vi "Main.vi"() -> ()   [LabVIEW 2021] (continued)
                w2497 = T9 9 items=["刷新间隔", "波特率", "布尔1设置项", "布尔2设置项", "布尔3设置项", "布尔4设置项", "布尔5设置项", "显控1设置", "显控2设置", "显控3设置", "显控4设置", "显控5设置", "显控6设置", "显控7设置", "显控8设置", "显控9设置", "显控10设置", "显控11设置", "显控12设置", "设控1设置", "设控2设置", "设控3设置", "设控4设置", "设控5设置", "设控6设置", "设控7设置", "设控8设置", "曲线1设置", "曲线2设置", "曲线3设置", "曲线4设置", "曲线5设置", "曲线6设置", "曲线7设置", "曲线8设置", "曲线9设置", "曲线10设置", "曲线11设置", "曲线12设置", "曲线13设置", "曲线14设置", "曲线15设置", "曲线16设置", "ID值"] ("DataInitDef")
                w2496 = T9 10 items=["刷新间隔", "波特率", "布尔1设置项", "布尔2设置项", "布尔3设置项", "布尔4设置项", "布尔5设置项", "显控1设置", "显控2设置", "显控3设置", "显控4设置", "显控5设置", "显控6设置", "显控7设置", "显控8设置", "显控9设置", "显控10设置", "显控11设置", "显控12设置", "设控1设置", "设控2设置", "设控3设置", "设控4设置", "设控5设置", "设控6设置", "设控7设置", "设控8设置", "曲线1设置", "曲线2设置", "曲线3设置", "曲线4设置", "曲线5设置", "曲线6设置", "曲线7设置", "曲线8设置", "曲线9设置", "曲线10设置", "曲线11设置", "曲线12设置", "曲线13设置", "曲线14设置", "曲线15设置", "曲线16设置", "ID值"] ("DataInitDef")
                w2495 = T9 11 items=["刷新间隔", "波特率", "布尔1设置项", "布尔2设置项", "布尔3设置项", "布尔4设置项", "布尔5设置项", "显控1设置", "显控2设置", "显控3设置", "显控4设置", "显控5设置", "显控6设置", "显控7设置", "显控8设置", "显控9设置", "显控10设置", "显控11设置", "显控12设置", "设控1设置", "设控2设置", "设控3设置", "设控4设置", "设控5设置", "设控6设置", "设控7设置", "设控8设置", "曲线1设置", "曲线2设置", "曲线3设置", "曲线4设置", "曲线5设置", "曲线6设置", "曲线7设置", "曲线8设置", "曲线9设置", "曲线10设置", "曲线11设置", "曲线12设置", "曲线13设置", "曲线14设置", "曲线15设置", "曲线16设置", "ID值"] ("DataInitDef")
                w2494 = T9 18 items=["刷新间隔", "波特率", "布尔1设置项", "布尔2设置项", "布尔3设置项", "布尔4设置项", "布尔5设置项", "显控1设置", "显控2设置", "显控3设置", "显控4设置", "显控5设置", "显控6设置", "显控7设置", "显控8设置", "显控9设置", "显控10设置", "显控11设置", "显控12设置", "设控1设置", "设控2设置", "设控3设置", "设控4设置", "设控5设置", "设控6设置", "设控7设置", "设控8设置", "曲线1设置", "曲线2设置", "曲线3设置", "曲线4设置", "曲线5设置", "曲线6设置", "曲线7设置", "曲线8设置", "曲线9设置", "曲线10设置", "曲线11设置", "曲线12设置", "曲线13设置", "曲线14设置", "曲线15设置", "曲线16设置", "ID值"] ("DataInitDef")
                w2493 = T9 12 items=["刷新间隔", "波特率", "布尔1设置项", "布尔2设置项", "布尔3设置项", "布尔4设置项", "布尔5设置项", "显控1设置", "显控2设置", "显控3设置", "显控4设置", "显控5设置", "显控6设置", "显控7设置", "显控8设置", "显控9设置", "显控10设置", "显控11设置", "显控12设置", "设控1设置", "设控2设置", "设控3设置", "设控4设置", "设控5设置", "设控6设置", "设控7设置", "设控8设置", "曲线1设置", "曲线2设置", "曲线3设置", "曲线4设置", "曲线5设置", "曲线6设置", "曲线7设置", "曲线8设置", "曲线9设置", "曲线10设置", "曲线11设置", "曲线12设置", "曲线13设置", "曲线14设置", "曲线15设置", "曲线16设置", "ID值"] ("DataInitDef")
                w2504 = T9 7 items=["刷新间隔", "波特率", "布尔1设置项", "布尔2设置项", "布尔3设置项", "布尔4设置项", "布尔5设置项", "显控1设置", "显控2设置", "显控3设置", "显控4设置", "显控5设置", "显控6设置", "显控7设置", "显控8设置", "显控9设置", "显控10设置", "显控11设置", "显控12设置", "设控1设置", "设控2设置", "设控3设置", "设控4设置", "设控5设置", "设控6设置", "设控7设置", "设控8设置", "曲线1设置", "曲线2设置", "曲线3设置", "曲线4设置", "曲线5设置", "曲线6设置", "曲线7设置", "曲线8设置", "曲线9设置", "曲线10设置", "曲线11设置", "曲线12设置", "曲线13设置", "曲线14设置", "曲线15设置", "曲线16设置", "ID值"] ("DataInitDef")
                w2499 = T9 13 items=["刷新间隔", "波特率", "布尔1设置项", "布尔2设置项", "布尔3设置项", "布尔4设置项", "布尔5设置项", "显控1设置", "显控2设置", "显控3设置", "显控4设置", "显控5设置", "显控6设置", "显控7设置", "显控8设置", "显控9设置", "显控10设置", "显控11设置", "显控12设置", "设控1设置", "设控2设置", "设控3设置", "设控4设置", "设控5设置", "设控6设置", "设控7设置", "设控8设置", "曲线1设置", "曲线2设置", "曲线3设置", "曲线4设置", "曲线5设置", "曲线6设置", "曲线7设置", "曲线8设置", "曲线9设置", "曲线10设置", "曲线11设置", "曲线12设置", "曲线13设置", "曲线14设置", "曲线15设置", "曲线16设置", "ID值"] ("DataInitDef")
                w2503 = T9 14 items=["刷新间隔", "波特率", "布尔1设置项", "布尔2设置项", "布尔3设置项", "布尔4设置项", "布尔5设置项", "显控1设置", "显控2设置", "显控3设置", "显控4设置", "显控5设置", "显控6设置", "显控7设置", "显控8设置", "显控9设置", "显控10设置", "显控11设置", "显控12设置", "设控1设置", "设控2设置", "设控3设置", "设控4设置", "设控5设置", "设控6设置", "设控7设置", "设控8设置", "曲线1设置", "曲线2设置", "曲线3设置", "曲线4设置", "曲线5设置", "曲线6设置", "曲线7设置", "曲线8设置", "曲线9设置", "曲线10设置", "曲线11设置", "曲线12设置", "曲线13设置", "曲线14设置", "曲线15设置", "曲线16设置", "ID值"] ("DataInitDef")
                w2500 = T9 15 items=["刷新间隔", "波特率", "布尔1设置项", "布尔2设置项", "布尔3设置项", "布尔4设置项", "布尔5设置项", "显控1设置", "显控2设置", "显控3设置", "显控4设置", "显控5设置", "显控6设置", "显控7设置", "显控8设置", "显控9设置", "显控10设置", "显控11设置", "显控12设置", "设控1设置", "设控2设置", "设控3设置", "设控4设置", "设控5设置", "设控6设置", "设控7设置", "设控8设置", "曲线1设置", "曲线2设置", "曲线3设置", "曲线4设置", "曲线5设置", "曲线6设置", "曲线7设置", "曲线8设置", "曲线9设置", "曲线10设置", "曲线11设置", "曲线12设置", "曲线13设置", "曲线14设置", "曲线15设置", "曲线16设置", "ID值"] ("DataInitDef")
                w2502 = T9 16 items=["刷新间隔", "波特率", "布尔1设置项", "布尔2设置项", "布尔3设置项", "布尔4设置项", "布尔5设置项", "显控1设置", "显控2设置", "显控3设置", "显控4设置", "显控5设置", "显控6设置", "显控7设置", "显控8设置", "显控9设置", "显控10设置", "显控11设置", "显控12设置", "设控1设置", "设控2设置", "设控3设置", "设控4设置", "设控5设置", "设控6设置", "设控7设置", "设控8设置", "曲线1设置", "曲线2设置", "曲线3设置", "曲线4设置", "曲线5设置", "曲线6设置", "曲线7设置", "曲线8设置", "曲线9设置", "曲线10设置", "曲线11设置", "曲线12设置", "曲线13设置", "曲线14设置", "曲线15设置", "曲线16设置", "ID值"] ("DataInitDef")
                w2501 = T9 17 items=["刷新间隔", "波特率", "布尔1设置项", "布尔2设置项", "布尔3设置项", "布尔4设置项", "布尔5设置项", "显控1设置", "显控2设置", "显控3设置", "显控4设置", "显控5设置", "显控6设置", "显控7设置", "显控8设置", "显控9设置", "显控10设置", "显控11设置", "显控12设置", "设控1设置", "设控2设置", "设控3设置", "设控4设置", "设控5设置", "设控6设置", "设控7设置", "设控8设置", "曲线1设置", "曲线2设置", "曲线3设置", "曲线4设置", "曲线5设置", "曲线6设置", "曲线7设置", "曲线8设置", "曲线9设置", "曲线10设置", "曲线11设置", "曲线12设置", "曲线13设置", "曲线14设置", "曲线15设置", "曲线16设置", "ID值"] ("DataInitDef")
                n1889 = local read "控件配置文件"() -> (w2518:string[][])
                n1890 = local read "表格"() -> (w2517:string[][])
                n1891 = call "显示处理.vi"("项目"=w2500, "配置文件"=w2518, "表格"=w2517) -> ("显示"=→"显控9":string)  [unwired: 8 in]
                n1892 = call "显示处理.vi"("项目"=w2502, "配置文件"=w2518, "表格"=w2517) -> ("显示"=→"显控10":string)  [unwired: 8 in]
                n1893 = call "显示处理.vi"("项目"=w2503, "配置文件"=w2518, "表格"=w2517) -> ("显示"=→"显控8":string)  [unwired: 8 in]
                n1894 = call "显示处理.vi"("项目"=w2499, "配置文件"=w2518, "表格"=w2517) -> ("显示"=→"显控7":string)  [unwired: 8 in]
                n1895 = call "显示处理.vi"("项目"=w2501, "配置文件"=w2518, "表格"=w2517) -> ("显示"=→"显控11":string)  [unwired: 8 in]
                n1896 = call "显示处理.vi"("项目"=w2504, "配置文件"=w2518, "表格"=w2517) -> ("显示"=→"显控1":string)  [unwired: 8 in]
                n1897 = call "显示处理.vi"("项目"=w2497, "配置文件"=w2518, "表格"=w2517) -> ("显示"=→"显控3":string)  [unwired: 8 in]
                n1898 = call "显示处理.vi"("项目"=w2498, "配置文件"=w2518, "表格"=w2517) -> ("显示"=→"显控2":string)  [unwired: 8 in]
                n1899 = call "显示处理.vi"("项目"=w2496, "配置文件"=w2518, "表格"=w2517) -> ("显示"=→"显控4":string)  [unwired: 8 in]
                n1900 = call "显示处理.vi"("项目"=w2495, "配置文件"=w2518, "表格"=w2517) -> ("显示"=→"显控5":string)  [unwired: 8 in]
                n1901 = call "显示处理.vi"("项目"=w2494, "配置文件"=w2518, "表格"=w2517) -> ("显示"=→"显控12":string)  [unwired: 8 in]
                n1902 = call "显示处理.vi"("项目"=w2493, "配置文件"=w2518, "表格"=w2517) -> ("显示"=→"显控6":string)  [unwired: 8 in]
                n1903 = local read "控件配置文件"() -> (w2483:string[][])
                n1904 = local read "表格"() -> (w2484:string[][])
                n1905 = call "显示处理.vi"("项目"=w2485, "配置文件"=w2483, "表格"=w2484) -> ("显示"=w2482:string)  [unwired: 8 in]
                n1906 = call "显示处理.vi"("项目"=w2488, "配置文件"=w2483, "表格"=w2484) -> ("显示"=w2481:string)  [unwired: 8 in]
                n1907 = call "显示处理.vi"("项目"=w2487, "配置文件"=w2483, "表格"=w2484) -> ("显示"=w2480:string)  [unwired: 8 in]
                n1908 = call "显示处理.vi"("项目"=w2489, "配置文件"=w2483, "表格"=w2484) -> ("显示"=w2479:string)  [unwired: 8 in]
                n1909 = call "显示处理.vi"("项目"=w2490, "配置文件"=w2483, "表格"=w2484) -> ("显示"=w2478:string)  [unwired: 8 in]
                n1910 = call "显示处理.vi"("项目"=w2491, "配置文件"=w2483, "表格"=w2484) -> ("显示"=w2477:string)  [unwired: 8 in]
                n1911 = call "显示处理.vi"("项目"=w2492, "配置文件"=w2483, "表格"=w2484) -> ("显示"=w2476:string)  [unwired: 8 in]
                n1912 = call "显示处理.vi"("项目"=w2486, "配置文件"=w2483, "表格"=w2484) -> ("显示"=w2475:string)  [unwired: 8 in]
                n1913 = local write "设控6"(w2477) -> ()
                n1914 = local write "设控7"(w2476) -> ()
                n1915 = local write "设控1"(w2482) -> ()
                n1916 = local write "设控4"(w2479) -> ()
                n1917 = local write "设控8"(w2475) -> ()
                n1918 = local write "设控2"(w2481) -> ()
                n1919 = local write "设控3"(w2480) -> ()
                n1920 = local write "设控5"(w2478) -> ()
              }
            }
          }
        }
      }
      frame #3 {
        n1921 = disable-structure shown="启用" {
          frame Disabled {
          }
          frame Enabled {
          }
        }
      }
    }
    n1922 = Wait on Notification(notifier=w26) -> (error out=w27:errorcluster)  [unwired: 3 in, 3 out]
  }
  n1923 = Build Path(base path=w16, name or relative path="Config\\Config.ini" ("名称或相对路径")) -> (appended path=w15:path)
  n1924 = timed-loop {
    shift-right: [w2536] -> _
    shift-left: w24 -> [w2537]
    shift-right: [w2534] -> w3
    shift-left: errorcluster {"status"=FALSE, "code"=0, "source"=""} ("error constant") -> [w2535]
    tunnel: w15 -> [w2531]
    timing: w20 -> [_]
    timing-out: [_] -> w19
    shift-right: [w2529] -> w13
    shift-left: w10 -> [w2524]
    shift-right: [w2528] -> w12
    shift-left: w14 -> [w2530]
    tunnel: w7 -> [w2523]
    stop <- FALSE stop-if-true
    # "主程序通信VI状态机"
    n1925 = node-c288() -> ()  [unwired: 1 in, 1 out]
    n1926 = Increment(x="i1") -> (x+1=w2519:i32)
    n1927 = case shown="\"Process\"" w2537 {
      tunnel: [w2596 w2627 w2653 w2668 w2826 w2830 w2836] -> w2536
      tunnel: [w2597 FALSE ("停止循环？") FALSE ("停止循环？") FALSE ("停止循环？") TRUE ("停止循环？") FALSE ("停止循环？") FALSE ("布尔 2")] -> _
      tunnel: w2535 -> [_ w2640 w2659 _ w2823 w2832 w2837]
      tunnel: [w2590 w2638 w2650 _ w2825 w2831 w2837] -> w2534
      tunnel: "重新连接" -> [w2595 w2626 w2652 w2667 _ _ _]
      tunnel: w2519 -> [_ _ _ w2661 _ _ _]
      tunnel: w2531 -> [w2589 _ _ _ _ _ _]
      frame "Initialize", Default {
        w2591 = State."ERROR"  # 下一个状态
        w2597 = FALSE  # 停止循环？
        w2594 = State."ResetCAN"  # 下一个状态
        # "初始化－对应用程序进行初始化。"
        n1928 = Select(t=w2594, s=TRUE, f=State."Exit" ("下一个状态")) -> (s? t:f=w2592:T3)
        n1929 = flat-sequence {
          tunnel: w2589 -> [w2599]
          tunnel: [w2599] -> w2588
          tunnel: w2588 -> [w2609]
          tunnel: [w2611] -> w2590
          frame #0 {
            n1930 = for {
              N: 8 -> [_]
              i -> [w2601]
              n1931 = Add(x=81, y=w2601) -> (x+y=w2600:i32)
              n1932 = call "CAN Uninitialize.vi"("Channel"=w2600) -> ()  [unwired: 9 in, 2 out]
            }
          }
          frame #1 {
            w2603 = T9 1 items=["刷新间隔", "波特率", "布尔1设置项", "布尔2设置项", "布尔3设置项", "布尔4设置项", "布尔5设置项", "布尔6设置项", "布尔7设置项", "布尔8设置项", "显控1设置", "显控2设置", "显控3设置", "显控4设置", "显控5设置", "显控6设置", "显控7设置", "显控8设置", "显控9设置", "显控10设置", "显控11设置", "显控12设置", "设控1设置", "设控2设置", "设控3设置", "设控4设置", "设控5设置", "设控6设置", "设控7设置", "设控8设置", "曲线1设置", "曲线2设置", "曲线3设置", "曲线4设置", "曲线5设置", "曲线6设置", "曲线7设置", "曲线8设置", "曲线9设置", "曲线10设置", "曲线11设置", "曲线12设置", "曲线13设置", "曲线14设置", "曲线15设置", "曲线16设置", "曲线17设置", "曲线18设置", "曲线19设置", "曲线20设置", "曲线21设置", "曲线22设置", "曲线23设置", "曲线24设置", "曲线25设置", "曲线26设置", "曲线27设置", "曲线28设置", "曲线29设置", "曲线30设置", "曲线31设置", "曲线32设置", "曲线33设置", "曲线34设置", "曲线35设置", "曲线36设置", "曲线37设置", "曲线38设置", "曲线39设置", "曲线40设置", "曲线41设置", "曲线42设置", "曲线43设置", "曲线44设置", "曲线45设置", "曲线46设置", "曲线47设置", "曲线48设置", "曲线49设置", "曲线50设置", "曲线51设置", "曲线52设置", "曲线53设置", "曲线54设置", "曲线55设置", "曲线56设置", "曲线57设置", "曲线58设置", "曲线59设置", "曲线60设置", "曲线61设置", "曲线62设置", "曲线63设置", "曲线64设置", "ID值", "数据模式"] ("DataInitDef")
            w2604 = T9 0 items=["刷新间隔", "波特率", "布尔1设置项", "布尔2设置项", "布尔3设置项", "布尔4设置项", "布尔5设置项", "布尔6设置项", "布尔7设置项", "布尔8设置项", "显控1设置", "显控2设置", "显控3设置", "显控4设置", "显控5设置", "显控6设置", "显控7设置", "显控8设置", "显控9设置", "显控10设置", "显控11设置", "显控12设置", "设控1设置", "设控2设置", "设控3设置", "设控4设置", "设控5设置", "设控6设置", "设控7设置", "设控8设置", "曲线1设置", "曲线2设置", "曲线3设置", "曲线4设置", "曲线5设置", "曲线6设置", "曲线7设置", "曲线8设置", "曲线9设置", "曲线10设置", "曲线11设置", "曲线12设置", "曲线13设置", "曲线14设置", "曲线15设置", "曲线16设置", "曲线17设置", "曲线18设置", "曲线19设置", "曲线20设置", "曲线21设置", "曲线22设置", "曲线23设置", "曲线24设置", "曲线25设置", "曲线26设置", "曲线27设置", "曲线28设置", "曲线29设置", "曲线30设置", "曲线31设置", "曲线32设置", "曲线33设置", "曲线34设置", "曲线35设置", "曲线36设置", "曲线37设置", "曲线38设置", "曲线39设置", "曲线40设置", "曲线41设置", "曲线42设置", "曲线43设置", "曲线44设置", "曲线45设置", "曲线46设置", "曲线47设置", "曲线48设置", "曲线49设置", "曲线50设置", "曲线51设置", "曲线52设置", "曲线53设置", "曲线54设置", "曲线55设置", "曲线56设置", "曲线57设置", "曲线58设置", "曲线59设置", "曲线60设置", "曲线61设置", "曲线62设置", "曲线63设置", "曲线64设置", "ID值", "数据模式"] ("DataInitDef")
            w2606 = T12 0 items=["CONFIG"] ("Config Section")
            # "1、从配置文件中读取上一次的记录。"
            n1933 = call "Read ini.vi"("configuration file path"=w2609) -> ("数组"=w2605:string[][])  [unwired: 10 in]
            "配置文件" <- w2605
            n1934 = Index Array(array=w2605, index (row)=w2606, index (col)=w2604) -> (element=w2610:string)
            n1935 = Index Array(array=w2605, index (row)=w2606, index (col)=w2603) -> (element=w2608:string)
            n1936 = property on="刷新间隔" class="Str"("Value"=w2610) -> ()  [unwired: 2 in, 2 out]
            n1937 = Hexadecimal String To Number(string=w2608) -> (number=w2607:u32)  [unwired: 2 in, 1 out]
            n1938 = property on="波特率" class="Ring (严格)"("Value"=w2607) -> ()  [unwired: 2 in, 2 out]
          }
          frame #2 {
            # "2、初始化CAN"
            n1939 = while {
              tunnel: [w2621] -> w2611
              i -> [w2614]
              stop <- w2615 stop-if-true
              w2613 = u8 81 ("Channel")
              n1940 = Add(x=w2613, y=w2614) -> (x+y=w2612:i32)
              "CAN通道" <- w2612
              n1941 = call "CAN Initialize.vi"("Btr0Btr1"="波特率", "Channel"=w2612) -> ("error out"=w2621:errorcluster, "function return"=w2616:u32)  [unwired: 8 in]
              n1942 = Equal To 0?(x=w2616) -> (x = 0?=w2617:bool)
              n1943 = Greater?(x=w2613, y=7) -> (0:w2618:bool)
              n1944 = Or(x=w2618, y=w2617) -> (x .or. y?=w2615:bool)
            }
          }
        }
        n1945 = Select(t=w2591, s=w2595, f=w2592) -> (s? t:f=w2596:T3)
        n1946 = call <vilib>:"Application Directory.vi"() -> ("Application Directory"=w2587:path)
        n1947 = Path To String(path=w2587) -> (string=w2586:string)
        n1948 = Reverse String(1:w2586) -> (0:w2585:string)
        n1949 = Match Pattern(string=w2585, regular expression="\\" ("正则表达式")) -> (before substring=w2583:string)  [unwired: 1 in, 3 out]
        n1950 = Reverse String(1:w2583) -> (0:w2582:string)
        n1951 = property on="项目名" class="Str"("Caption.Text"=w2582) -> ()  [unwired: 2 in, 2 out]
      }
      frame "ResetCAN" {
        # "复位CAN模块，并读取CAN模块的状态"
        n1952 = local read "CAN通道"() -> (w2623:u8)
        n1953 = call "CAN Reset.vi"("error in (no error)"=w2640, "Channel"=w2623) -> ("error out"=w2639:errorcluster, "function return"=w2634:u32)  [unwired: 8 in]
        n1954 = call "CAN Get Status.vi"("error in (no error)"=w2639, "Channel"=w2623) -> ("error out"=w2638:errorcluster, "function return"=w2637:u32)  [unwired: 8 in]
        n1955 = Equal To 0?(x=w2634) -> (x = 0?=w2633:bool)
        n1956 = Equal To 0?(x=w2637) -> (x = 0?=w2632:bool)
        n1957 = And(x=w2633, y=w2632) -> (x .and. y?=w2624:bool)
        n1958 = Select(t=State."SetCAN" ("下一个状态"), s=w2624, f=State."ERROR" ("返回初始状态")) -> (s? t:f=w2630:T3)
        n1959 = Select(t=w2630, s=TRUE, f=State."Exit" ("返回初始状态")) -> (s? t:f=w2628:T3)
        n1960 = Select(t=State."ERROR" ("下一个状态"), s=w2626, f=w2628) -> (s? t:f=w2627:T3)
      }
      frame "SetCAN" {
        w2655 = State."ERROR"  # 下一个状态
        w2657 = State."Exit"  # 返回初始状态
        w2656 = State."Process"  # 初始状态
        # "设置CAN模块的参数"
        n1961 = local read "CAN通道"() -> (w2643:u8)
        n1962 = Select(t=w2656, s=TRUE, f=w2657) -> (s? t:f=w2654:T3)
        n1963 = call "CAN Get Value.vi"("BufferLength"=u32 4, "error in (no error)"=w2659, "Parameter"=u8 1, "Channel"=w2643) -> ("error out"=w2644:errorcluster)  [unwired: 4 in, 3 out]
        n1964 = Select(t=w2655, s=w2652, f=w2654) -> (s? t:f=w2653:T3)
        n1965 = call "CAN Set Value.vi"("BufferLength"=u32 1280, "error in (no error)"=w2644, "Parameter"=u8 3, "Channel"=w2643) -> ("error out"=w2645:errorcluster)  [unwired: 5 in, 2 out]
        n1966 = local read "ID"() -> (w2648:u32)
        n1967 = call "CAN Filter Messages.vi"("Mode"=u8 2, "error in (no error)"=w2645, "ToID"=w2648, "FromID"=w2648, "Channel"=w2643) -> ("error out"=w2650:errorcluster)  [unwired: 5 in, 1 out]
      }
      frame "Process" {
        w2662 = State."ERROR"  # 下一个状态
        w2665 = State."Exit"  # 返回初始状态
        w2666 = State."Process"  # 初始状态
        n1968 = stacked-sequence {
          tunnel: w2661 -> [_ _ w2754]
          frame #0 {
            n1969 = while {
              stop <- w2673 continue-if-true
              (unwired) TRUE ("y")
              n1970 = local read "CAN通道"() -> (w2671:u8)
              n1971 = local read "ID"() -> (w2672:u32)
              n1972 = call "CAN Read.vi"("Channel"=w2671) -> ("data"=w2675:u8[], "function return"=w2674:u32, "ID"=w2670:u32)  [unwired: 6 in, 2 out]
              n1973 = Equal To 0?(x=w2674) -> (x = 0?=w2673:bool)
              n1974 = Equal?(x=w2670, y=w2672) -> (x = y?=w2669:bool)
              n1975 = And(x=w2673, y=w2669) -> (x .and. y?=w2676:bool)
              n1976 = case shown="真" w2676 {
                tunnel: w2675 -> [_ w2704]
                tunnel: w2670 -> [_ w2693]
                frame False {
                  n1977 = local read "刷新间隔"() -> (w2683:string)
                  n1978 = Decimal String To Number(string=w2683) -> (number=w2682:i32)  [unwired: 2 in, 1 out]
                  n1979 = local read "错误计数器"() -> (w2684:u32)
                  n1980 = Multiply(x=w2682, y=2) -> (x*y=w2679:i32)
                  n1981 = Increment(x=w2684) -> (x+1=w2687:u32)
                  n1982 = Add(x=10, y=w2679) -> (x+y=w2678:i32)
                  n1983 = Greater?(x=w2687, y=w2678) -> (0:w2688:bool)
                  n1984 = Decrement(x=w2678) -> (x-1=w2680:i32)
                  n1985 = Greater?(x=w2684, y=w2680) -> (0:w2685:bool)
                  n1986 = Select(t=w2678, s=w2688, f=w2687) -> (s? t:f=→"错误计数器":u32)
                  n1987 = case shown="假" w2685 {
                    frame False {
                      n1988 = property on="通信状态" class="Str"("Value"="正常" ("通信状态")) -> ()  [unwired: 2 in, 2 out]
                      n1989 = property on="通信状态" class="Str"("Text.TextColor"=u32 65280 ("文本.文本颜色:文本颜色")) -> ()  [unwired: 2 in, 2 out]
                    }
                    frame True {
                      n1990 = property on="通信状态" class="Str"("Value"="错误" ("通信状态")) -> ()  [unwired: 2 in, 2 out]
                      n1991 = property on="通信状态" class="Str"("Text.TextColor"=u32 16711680 ("文本.文本颜色:文本颜色")) -> ()  [unwired: 2 in, 2 out]
                    }
                  }
                }
                frame True {
                  # "CRC验证码校验"
                  n1992 = Split 1D Array(array=w2704, index=6 ("索引")) -> (first subarray=w2694:u8[], second subarray=w2700:u8[])
                  n1993 = call "CRC_A965 .vi"("U8"=w2694) -> ("CRC-16"=w2697:u16)  [unwired: 10 in]
                  n1994 = Index Array(array=w2700, index=1 ("索引")) -> (element=w2701:u8)
                  n1995 = Index Array(array=w2700, index=0 ("索引")) -> (element=w2698:u8)
                  n1996 = Join Numbers(hi=w2701, lo=w2698) -> ((hi.lo)=w2696:u16)
                  n1997 = Equal?(x=w2697, y=w2696) -> (x = y?=w2695:bool)
                  n1998 = case shown="真" w2695 {
                    tunnel: w2694 -> [_ w2711]
                    tunnel: w2693 -> [_ w2705]
                    frame False {
                    }
                    frame True {
                      # "当收到的功能码为1时，写入表格"
                      n1999 = Index Array(array=w2711, index=0 ("索引")) -> (element=w2739:u8)
                      n2000 = Index Array(array=w2711, index=1 ("索引")) -> (element=w2728:u8)
                      n2001 = Index Array(array=w2711, index=2 ("索引")) -> (element=w2736:u8)
                      n2002 = Index Array(array=w2711, index=3 ("索引")) -> (element=w2726:u8)
                      n2003 = Index Array(array=w2711, index=4 ("索引")) -> (element=w2717:u8)
                      n2004 = Index Array(array=w2711, index=5 ("索引")) -> (element=w2714:u8)
                      n2005 = To Unsigned Word Integer(number=w2714) -> (unsigned 16bit integer=w2713:u16)
                      n2006 = To Unsigned Word Integer(number=w2726) -> (unsigned 16bit integer=w2725:u16)
                      n2007 = And(x=w2728, y=u8 15) -> (x .and. y?=w2724:u8)
                      n2008 = Logical Shift(y=i16 -4, x=w2728) -> (x << y=w2727:u8)
                      n2009 = Logical Shift(y=i16 8, x=w2713) -> (x << y=w2715:u16)
                      n2010 = To Unsigned Word Integer(number=w2724) -> (unsigned 16bit integer=w2723:u16)
                      n2011 = And(x=w2727, y=u16 3) -> (x .and. y?=w2721:u16)
                      n2012 = Logical Shift(y=i16 8, x=w2725) -> (x << y=w2732:u16)
                      n2013 = Add(x=w2717, y=w2715) -> (x+y=w2712:u16)
                      n2014 = Add(x=w2736, y=w2732) -> (x+y=w2708:u16)
                      n2015 = Logical Shift(y=i16 8, x=w2723) -> (x << y=w2730:u16)
                      n2016 = To Unsigned Long Integer(number=w2712) -> (unsigned 32bit integer=w2710:u32)
                      n2017 = Add(x=w2739, y=w2730) -> (x+y=w2735:u16)
                      n2018 = Logical Shift(y=i16 16, x=w2710) -> (x << y=w2706:u32)
                      n2019 = Equal?(x=w2721, y=u16 1) -> (x = y?=w2722:bool)
                      n2020 = Add(x=w2708, y=w2706) -> (x+y=w2707:u32)
                      n2021 = case shown="真" w2722 {
                        tunnel: w2735 -> [_ w2748]
                        tunnel: w2707 -> [_ w2747]
                        tunnel: w2705 -> [_ w2746]
                        frame False {
                        }
                        frame True {
                          n2022 = Build Array(w2748, w2747, w2746) -> (w2745:u32[])
                          n2023 = local read "CANBURF"() -> (w2744:u32[][])
                          n2024 = local write "错误计数器"(u32 0 ("数值 2")) -> ()
                          n2025 = call "收到的数据排序V2.vi"("BUF"=w2744, "输入数据"=w2745) -> ("BUF OUT"=w2743:u32[][])  [unwired: 7 in]
                          n2026 = local write "CANBURF"(w2743) -> ()
                        }
                      }
                    }
                  }
                }
              }
            }
          }
          frame #1 {
            n2027 = event shown="[1] \"要发送的数据\": 值改变" {
              selector: _ -> [_ _]
              dyn-events: _ -> [_ _]
              timeout: 0 -> [_ _]
              event Timeout {
                n2028 = event-data() -> ()  [unwired: 1 in, 3 out]
              }
              event "要发送的数据": Value Change {
                # "写入命令VI"
                n2029 = event-data() -> ()  [unwired: 1 in, 6 out]
                n2030 = local read "ID"() -> (w2751:u32)
                n2031 = property on="要发送的数据" class="Clust (严格)"() -> ("Value"=w2753:cluster{"地址":u16, "数据":i32, "行数":i32, "ID":i32})  [unwired: 2 in, 2 out]
                n2032 = local read "CAN通道"() -> (w2752:u8)
                n2033 = call "数据写入.vi"("CAN通道"=w2752, "ID"=w2751, "簇"=w2753) -> ()  [unwired: 9 in]
              }
            }
          }
          frame #2 {
            n2034 = Decimal String To Number(string="刷新间隔") -> (number=w2760:i32)  [unwired: 2 in, 1 out]
            n2035 = Equal To 0?(x=w2760) -> (x = 0?=w2757:bool)
            n2036 = Select(t=1, s=w2757, f=w2760) -> (s? t:f=w2758:i32)
            n2037 = Quotient & Remainder(x=w2754, y=w2758) -> (x-y*floor(x/y)=w2756:i32)  [unwired: 1 out]
            n2038 = Equal To 0?(x=w2756) -> (x = 0?=w2755:bool)
            n2039 = case shown="真" w2755 {
              frame False {
              }
              frame True {
                # "本框架为CAN通信主要框架，实现每隔指定的时间对参数列表中的参数进行循环发送和读取"
                n2040 = local read "表格"() -> (w2764:string[][])
                n2041 = property on="循环指针" class="DigNum (严格)"() -> ("Value"=w2763:u16)  [unwired: 2 in, 2 out]
                n2042 = disable-structure shown="禁用" {
                  disable-tunnel: w2764 -> [w2777 _]
                  disable-tunnel: w2763 -> [w2776 _]
                  frame Disabled {
                    n2043 = Index Array(array=w2777, index (row)=w2776, index (col)=7 ("禁用的索引 (列)")) -> (element=w2771:string)
                    n2044 = Hexadecimal String To Number(string=w2771) -> (number=w2770:u32)  [unwired: 2 in, 1 out]
                    n2045 = Equal?(x=w2771, y="") -> (x = y?=w2773:bool)
                    n2046 = Select(s=w2773, f=w2770) -> (s? t:f=→"运行ID":u32)  [unwired: 1 in]
                  }
                  frame Enabled {
                  }
                }
                n2047 = Index Array(array=w2764, index (row)=w2763, index (col)=0 ("禁用的索引 (列)")) -> (element=w2767:string)
                n2048 = Increment(x=w2763) -> (x+1=→"循环指针":u16)
                n2049 = local read "ID"() -> (w2762:u32)
                n2050 = Equal?(x=w2767, y="") -> (x = y?=w2765:bool)
                n2051 = case shown="真" w2765 {
                  tunnel: w2764 -> [w2781 _]
                  tunnel: w2763 -> [w2780 _]
                  tunnel: w2762 -> [w2779 _]
                  frame False {
                    # "如果下一行的第0列没有任何数据，则认为本表已经循环完毕。将指针回零重新下一轮的循环123456"
                    n2052 = local read "CAN通道"() -> (w2778:u8)
                    n2053 = call "循环读取命令.vi"("循环指针"=w2780, "表格"=w2781, "ID"=w2779, "CAN通道"=w2778) -> ()  [unwired: 8 in]
                  }
                  frame True {
                    # "如果下一行的第0列没有任何数据，则认为本表已经循环完毕。将指针回零重新下一轮的循环"
                    n2054 = stacked-sequence {
                      frame #0 {
                        n2055 = Tick Count (ms)() -> (millisecond timer value=w2783:u32)
                        n2056 = feedback-in #1(w2783) -> ()
                        n2057 = feedback #1() -> (w2784:u32)  [unwired: 1 in]
                        n2058 = Subtract(x=w2783, y=w2784) -> (x-y=w2785:u32)
                        n2059 = Divide(x=w2785, y=1000) -> (x/y=w2787:dbl)
                        n2060 = Number To Fractional String(number=w2787, precision (6)=i16 3 ("精度(6)")) -> (F-format string=w2786:string)  [unwired: 2 in]
                        n2061 = property on="轮询一次周期" class="Str"("Value"=w2786) -> ()  [unwired: 2 in, 2 out]
                      }
                      frame #1 {
                        n2062 = flat-sequence {
                          frame #0 {
                            # "波形记录"
                            n2063 = local read "控件配置文件"() -> (w2789:string[][])
                            n2064 = local read "表格"() -> (w2790:string[][])
                            n2065 = call "波形记录处理V2.vi"("控件配置文件"=w2789, "表格"=w2790) -> ("曲线数量"=w2791:u16, "曲线名称"=w2792:string[], "波形图"=w2793:dynamicdata)  [unwired: 7 in]
                            n2066 = case shown="真" "清除历史记录" {
                              frame False {
                              }
                              frame True {
                                n2067 = property on="波形图表" class="WFChart (严格)"("History Data"=dynamicdata[] [] ("历史数据")) -> ()  [unwired: 2 in, 2 out]
                              }
                            }
                            n2068 = feedback #2() -> (w2801:u16)  [unwired: 1 in]
                            n2069 = feedback-in #2(w2791) -> ()
                            n2070 = feedback #3() -> (w2797:string[])  [unwired: 1 in]
                            n2071 = feedback-in #3(w2792) -> ()
                            n2072 = case shown="真" "记录波形更新" {
                              tunnel: w2793 -> [_ w2810]
                              frame False {
                              }
                              frame True {
                                "波形图表" <- w2810
                              }
                            }
                            n2073 = Equal To 0?(x=w2791) -> (x = 0?=w2799:bool)
                            n2074 = Not Equal?(x=w2791, y=w2801) -> (x != y?=w2796:bool)
                            n2075 = Not Equal?(x=w2792, y=w2797) -> (x != y?=w2795:bool)
                            n2076 = Or(x=w2796, y=w2795) -> (x .or. y?=w2794:bool)
                            n2077 = case shown="真" w2794 {
                              tunnel: w2792 -> [_ w2811]
                              tunnel: w2791 -> [_ w2812]
                              frame False {
                              }
                              frame True {
                                n2078 = stacked-sequence {
                                tunnel: w2812 -> [w2813 _]
                                tunnel: w2811 -> [_ w2817]
                                frame #0 {
                                n2079 = disable-structure shown="禁用" {
                                disable-tunnel: w2813 -> [w2816 _]
                                frame Disabled {
                                n2080 = Greater Than 0?(x=w2816) -> (x > 0?=w2815:bool)
                                n2081 = property on="波形图表" class="WFChart (严格)"("LegNumRows"=w2816, "Legend Visible"=w2815, "Dig Display(s) Visible"=FALSE ("数字显示可见"), "LegPlotMin"=w2816) -> ()  [unwired: 2 in, 2 out]
                                }
                                frame Enabled {
                                }
                                }
                                }
                                frame #1 {
                                n2082 = for "For循环" {
                                tunnel: w2817 -> [w2819] mode=indexing
                                i -> [w2820]
                                n2083 = call "字符串比对X.vi"("字符串"=w2819) -> ("布尔"=w2818:bool)  [unwired: 10 in]
                                n2084 = property on="波形图表" class="WFChart (严格)"("Active Plot"=w2820, "Plot.Plot Name"=w2819, "Plot.Visible?"=w2818) -> ()  [unwired: 2 in, 2 out]
                                }
                                }
                                }
                              }
                            }
                            n2085 = feedback #4() -> (w2800:bool)  [unwired: 1 in]
                            n2086 = feedback-in #4(w2794) -> ()
                            n2087 = disable-structure shown="禁用" {
                              disable-tunnel: w2800 -> [w2806 _]
                              disable-tunnel: w2799 -> [w2805 _]
                              disable-tunnel: w2794 -> [w2804 _]
                              frame Disabled {
                                n2088 = Not Equal?(x=w2806, y=w2804) -> (x != y?=w2803:bool)
                                n2089 = case shown="真" w2803 {
                                frame False {
                                }
                                frame True {
                                n2090 = property on="波形图表" class="WFChart (严格)"("Dig Display(s) Visible"=TRUE) -> ()  [unwired: 2 in, 2 out]
                                }
                                }
                                n2091 = case shown="真" w2805 {
                                frame False {
                                }
                                frame True {
                                n2092 = property on="波形图表" class="WFChart (严格)"("Dig Display(s) Visible"=FALSE ("数字显示可见")) -> ()  [unwired: 2 in, 2 out]
                                }
                                }
                              }
                              frame Enabled {
                              }
                            }
                          }
                        }
                      }
                      frame #2 {
                        n2093 = property on="循环指针" class="DigNum (严格)"("Value"=u16 0 ("循环指针")) -> ()  [unwired: 2 in, 2 out]
                      }
                    }
                  }
                }
              }
            }
          }
        }
        n2094 = Select(t=w2666, s=TRUE, f=w2665) -> (s? t:f=w2664:T3)
        n2095 = Select(t=w2662, s=w2667, f=w2664) -> (s? t:f=w2668:T3)
      }
      frame "Exit" {
        w2826 = State."STOP"  # （下一个状态）
        # "退出－退出应用程序。"
        n2096 = local read "CAN通道"() -> (w2822:u8)
        n2097 = call "CAN Uninitialize.vi"("error in (no error)"=w2823, "Channel"=w2822) -> ("error out"=w2825:errorcluster)  [unwired: 8 in, 1 out]
      }
      frame "ERROR" {
        w2830 = State."Initialize"  # 初始状态
        n2098 = local read "CAN通道"() -> (w2828:u8)
        n2099 = call "CAN Uninitialize.vi"("error in (no error)"=w2832, "Channel"=w2828) -> ("error out"=w2833:errorcluster)  [unwired: 8 in, 1 out]
        n2100 = call <vilib>:"Simple Error Handler.vi"("error code (no error:0)"=0, "error in (no error)"=w2833) -> ("error out"=w2831:errorcluster)  [unwired: 3 in, 4 out]
        n2101 = Wait (ms)(milliseconds to wait=u32 10 ("等待时间（毫秒）")) -> ()  [unwired: 1 out]
      }
      frame "STOP" {
        w2836 = State."STOP"  # （未用值）
      }
    }
    n2102 = event shown="[1] \"波特率\", \"刷新间隔\", \"布控1设置\", \"显控1设置\", \"显控2设置\", \"显控3设置\", \"显控4设置\", \"显控5设置\", \"显控6设置\", \"显控7设置\", \"显控8设置\", \"显控9设置\", \"显控10设置\", \"显控11设置\", \"显控12设置\", \"布控2设置\", \"布控3设置\", \"布控4设置\", \"设控设置 1\", \"设控设置 2\", \"设控设置 3\", \"设控设置 4\", \"设控设置 5\", \"设控设置 6\", \"设控设置 7\", \"设控设置 8\", \"曲线1设置\", \"曲线2设置\", \"曲线3设置\", \"曲线4设置\", \"曲线5设置\", \"曲线6设置\", \"曲线7设置\", \"曲线8设置\", \"ID\", \"布控5设置\", \"曲线9设置\", \"曲线10设置\", \"曲线11设置\", \"曲线12设置\", \"曲线13设置\", \"曲线14设置\", \"曲线15设置\", \"曲线16设置\", \"数据模式\", \"布控6设置\", \"布控7设置\", \"布控8设置\", \"曲线17设置\", \"曲线18设置\", \"曲线19设置\", \"曲线20设置\", \"曲线21设置\", \"曲线22设置\", \"曲线23设置\", \"曲线24设置\", \"曲线25设置\", \"曲线26设置\", \"曲线27设置\", \"曲线28设置\", \"曲线29设置\", \"曲线30设置\", \"曲线31设置\", \"曲线32设置\", \"曲线33设置\", \"曲线34设置\", \"曲线35设置\", \"曲线36设置\", \"曲线37设置\", \"曲线38设置\", \"曲线39设置\", \"曲线40设置\", \"曲线41设置\", \"曲线42设置\", \"曲线43设置\", \"曲线44设置\", \"曲线45设置\", \"曲线46设置\", \"曲线47设置\", \"曲线48设置\", \"曲线49设置\", \"曲线50设置\", \"曲线51设置\", \"曲线52设置\", \"曲线53设置\", \"曲线54设置\", \"曲线55设置\", \"曲线56设置\", \"曲线57设置\", \"曲线58设置\", \"曲线59设置\", \"曲线60设置\", \"曲线61设置\", \"曲线62设置\", \"曲线63设置\", \"曲线64设置\": 值改变" {
      selector: _ -> [_ _]
      dyn-events: _ -> [_ _]
      timeout: 0 -> [_ _]
      tunnel: w2531 -> [_ w2552]
      tunnel: w2523 -> [_ w2549]
      event Timeout {
        n2103 = event-data() -> ()  [unwired: 1 in, 3 out]
      }
      event "波特率", "刷新间隔", "布控1设置", "显控1设置", "显控2设置", "显控3设置", "显控4设置", "显控5设置", "显控6设置", "显控7设置", "显控8设置", "显控9设置", "显控10设置", "显控11设置", "显控12设置", "布控2设置", "布控3设置", "布控4设置", "设控设置 1", "设控设置 2", "设控设置 3", "设控设置 4", "设控设置 5", "设控设置 6", "设控设置 7", "设控设置 8", "曲线1设置", "曲线2设置", "曲线3设置", "曲线4设置", "曲线5设置", "曲线6设置", "曲线7设置", "曲线8设置", "ID", "布控5设置", "曲线9设置", "曲线10设置", "曲线11设置", "曲线12设置", "曲线13设置", "曲线14设置", "曲线15设置", "曲线16设置", "数据模式", "布控6设置", "布控7设置", "布控8设置", "曲线17设置", "曲线18设置", "曲线19设置", "曲线20设置", "曲线21设置", "曲线22设置", "曲线23设置", "曲线24设置", "曲线25设置", "曲线26设置", "曲线27设置", "曲线28设置", "曲线29设置", "曲线30设置", "曲线31设置", "曲线32设置", "曲线33设置", "曲线34设置", "曲线35设置", "曲线36设置", "曲线37设置", "曲线38设置", "曲线39设置", "曲线40设置", "曲线41设置", "曲线42设置", "曲线43设置", "曲线44设置", "曲线45设置", "曲线46设置", "曲线47设置", "曲线48设置", "曲线49设置", "曲线50设置", "曲线51设置", "曲线52设置", "曲线53设置", "曲线54设置", "曲线55设置", "曲线56设置", "曲线57设置", "曲线58设置", "曲线59设置", "曲线60设置", "曲线61设置", "曲线62设置", "曲线63设置", "曲线64设置": Value Change {
        # "参数保存。当有更多的参数需要保存时，在此框图中增加事件触发和相应的元素"
        n2104 = event-data() -> ()  [unwired: 1 in, 3 out]
        n2105 = property on="刷新间隔" class="Str"() -> ("Label.Text"=w2558:string)  [unwired: 2 in, 2 out]
        n2106 = property on="波特率" class="Ring (严格)"() -> ("Value"=w2559:u16)  [unwired: 2 in, 2 out]
        n2107 = property on="波特率" class="Ring (严格)"() -> ("Label.Text"=w2556:string)  [unwired: 2 in, 2 out]
        n2108 = property on="刷新间隔" class="Str"() -> ("Value"=w2557:string)  [unwired: 2 in, 2 out]
        n2109 = Number To Hexadecimal String(2:w2559) -> (0:w2555:string)  [unwired: 1 in]
        n2110 = Build Array(w2558, w2557) -> (w2551:string[])
        n2111 = Build Array(w2556, w2555) -> (w2550:string[])
        n2112 = Build Array(w2551, w2550) -> (w2553:string[][])
        n2113 = call "Write ini.vi"("configuration file path"=w2552, "数组"=w2553, "段"="CONFIG" ("元素")) -> ()  [unwired: 9 in]
        n2114 = stacked-sequence {
          tunnel: w2549 -> [_ _ w2578]
          frame #0 {
            w2560 = T9 94 items=["刷新间隔", "波特率", "布尔1设置项", "布尔2设置项", "布尔3设置项", "布尔4设置项", "布尔5设置项", "布尔6设置项", "布尔7设置项", "布尔8设置项", "显控1设置", "显控2设置", "显控3设置", "显控4设置", "显控5设置", "显控6设置", "显控7设置", "显控8设置", "显控9设置", "显控10设置", "显控11设置", "显控12设置", "设控1设置", "设控2设置", "设控3设置", "设控4设置", "设控5设置", "设控6设置", "设控7设置", "设控8设置", "曲线1设置", "曲线2设置", "曲线3设置", "曲线4设置", "曲线5设置", "曲线6设置", "曲线7设置", "曲线8设置", "曲线9设置", "曲线10设置", "曲线11设置", "曲线12设置", "曲线13设置", "曲线14设置", "曲线15设置", "曲线16设置", "曲线17设置", "曲线18设置", "曲线19设置", "曲线20设置", "曲线21设置", "曲线22设置", "曲线23设置", "曲线24设置", "曲线25设置", "曲线26设置", "曲线27设置", "曲线28设置", "曲线29设置", "曲线30设置", "曲线31设置", "曲线32设置", "曲线33设置", "曲线34设置", "曲线35设置", "曲线36设置", "曲线37设置", "曲线38设置", "曲线39设置", "曲线40设置", "曲线41设置", "曲线42设置", "曲线43设置", "曲线44设置", "曲线45设置", "曲线46设置", "曲线47设置", "曲线48设置", "曲线49设置", "曲线50设置", "曲线51设置", "曲线52设置", "曲线53设置", "曲线54设置", "曲线55设置", "曲线56设置", "曲线57设置", "曲线58设置", "曲线59设置", "曲线60设置", "曲线61设置", "曲线62设置", "曲线63设置", "曲线64设置", "ID值", "数据模式"] ("DataInitDef")
            n2115 = local read "ID"() -> (w2562:u32)
            n2116 = Number To Hexadecimal String(2:w2562) -> (0:w2561:string)  [unwired: 1 in]
            n2117 = invoke on="控件配置文件" class="Tbl (严格)" method="Set Cell Value"("X Index"=1 ("X索引"), "Y Index"=w2560, "Value"=w2561) -> ()  [unwired: 3 in, 6 out]
            n2118 = invoke on="控件配置文件" class="Tbl (严格)" method="Set Cell Value"("X Index"=0 ("X索引"), "Y Index"=w2560, "Value"="ID" ("值")) -> ()  [unwired: 3 in, 6 out]
          }
          frame #1 {
            w2566 = T9 95 items=["刷新间隔", "波特率", "布尔1设置项", "布尔2设置项", "布尔3设置项", "布尔4设置项", "布尔5设置项", "布尔6设置项", "布尔7设置项", "布尔8设置项", "显控1设置", "显控2设置", "显控3设置", "显控4设置", "显控5设置", "显控6设置", "显控7设置", "显控8设置", "显控9设置", "显控10设置", "显控11设置", "显控12设置", "设控1设置", "设控2设置", "设控3设置", "设控4设置", "设控5设置", "设控6设置", "设控7设置", "设控8设置", "曲线1设置", "曲线2设置", "曲线3设置", "曲线4设置", "曲线5设置", "曲线6设置", "曲线7设置", "曲线8设置", "曲线9设置", "曲线10设置", "曲线11设置", "曲线12设置", "曲线13设置", "曲线14设置", "曲线15设置", "曲线16设置", "曲线17设置", "曲线18设置", "曲线19设置", "曲线20设置", "曲线21设置", "曲线22设置", "曲线23设置", "曲线24设置", "曲线25设置", "曲线26设置", "曲线27设置", "曲线28设置", "曲线29设置", "曲线30设置", "曲线31设置", "曲线32设置", "曲线33设置", "曲线34设置", "曲线35设置", "曲线36设置", "曲线37设置", "曲线38设置", "曲线39设置", "曲线40设置", "曲线41设置", "曲线42设置", "曲线43设置", "曲线44设置", "曲线45设置", "曲线46设置", "曲线47设置", "曲线48设置", "曲线49设置", "曲线50设置", "曲线51设置", "曲线52设置", "曲线53设置", "曲线54设置", "曲线55设置", "曲线56设置", "曲线57设置", "曲线58设置", "曲线59设置", "曲线60设置", "曲线61设置", "曲线62设置", "曲线63设置", "曲线64设置", "ID值", "数据模式"] ("DataInitDef")
            n2119 = local read "数据模式"() -> (w2567:bool)
            n2120 = Boolean To (0,1)(Boolean=w2567) -> (0, 1=w2568:i16)
            n2121 = Number To Hexadecimal String(2:w2568) -> (0:w2569:string)  [unwired: 1 in]
            n2122 = invoke on="控件配置文件" class="Tbl (严格)" method="Set Cell Value"("X Index"=1 ("X索引"), "Y Index"=w2566, "Value"=w2569) -> ()  [unwired: 3 in, 6 out]
            n2123 = invoke on="控件配置文件" class="Tbl (严格)" method="Set Cell Value"("X Index"=0 ("X索引"), "Y Index"=w2566, "Value"="数据模式" ("值")) -> ()  [unwired: 3 in, 6 out]
          }
          frame #2 {
            n2124 = property on="控件配置文件" class="Tbl (严格)"() -> ("Value"=w2576:string[][])  [unwired: 2 in, 2 out]
            n2125 = Array To Spreadsheet String(array=w2576, 3:"%s" ("格式字符串")) -> (spreadsheet string=w2575:string)  [unwired: 1 in]
            n2126 = Write to Text File(file (use dialog)=w2578, text=w2575) -> (refnum out=w2574:refnum<file>, error out=w2573:errorcluster)  [unwired: 2 in, 1 out]
            n2127 = Close File(refnum=w2574, error in=w2573) -> ()  [unwired: 2 out]
          }
        }
      }
    }
    n2128 = local write "i1"(w2519) -> ()
    n2129 = Quotient & Remainder(x=w2519, y=20) -> (x-y*floor(x/y)=w2526:i32)  [unwired: 1 out]
    n2130 = event shown="[1] \"退出\": 值改变" {
      selector: _ -> [_ _]
      dyn-events: _ -> [_ _]
      timeout: 0 -> [_ _]
      event Timeout {
        n2131 = event-data() -> ()  [unwired: 1 in, 3 out]
      }
      event "退出": Value Change {
        n2132 = event-data() -> ()  [unwired: 1 in, 6 out]
        n2133 = Two Button Dialog(message="确定退出" ("消息")) -> (T button?=w2539:bool)  [unwired: 2 in]
        n2134 = case shown="真" w2539 {
          frame False {
          }
          frame True {
            n2135 = local read "CAN通道"() -> (w2540:u8)
            n2136 = Quit LabVIEW(quit? (T)=TRUE ("退出？(T)")) -> ()
            n2137 = call "CAN Uninitialize.vi"("Channel"=w2540) -> ()  [unwired: 9 in, 2 out]
          }
        }
      }
    }
    n2138 = Equal To 0?(x=w2526) -> (x = 0?=w2525:bool)
    n2139 = case shown="真" w2525 {
      tunnel: w2524 -> [w2543 w2547]
      tunnel: w2530 -> [w2542 w2546]
      tunnel: [w2543 w2545] -> w2529
      tunnel: [w2542 w2544] -> w2528
      frame False {
      }
      frame True {
        # "每20ms发送一个通知启动界面程序"
        n2140 = call "Error_mx.vi"() -> ()  [unwired: 12 in]
        n2141 = Send Notification(notification="RUN" ("通知"), notifier=w2547, error in (no error)=w2546) -> (notifier out=w2545:refnum<notifier>, error out=w2544:errorcluster)
      }
    }
    n2142 = node-c288() -> ()  [unwired: 1 in, 1 out]
  }
  n2143 = node-c288(w19) -> ()  [unwired: 1 out]
  n2144 = local read "CAN通道"() -> (w1:u8)
  n2145 = local read "CAN通道"() -> (w2:u8)
  n2146 = Release Notifier(notifier=w13, error in (no error)=w12) -> (error out=w4:errorcluster)  [unwired: 1 in, 2 out]
  n2147 = call "CAN Uninitialize.vi"("error in (no error)"=w3, "Channel"=w1) -> ("error out"=w21:errorcluster)  [unwired: 8 in, 1 out]
  n2148 = call "CAN Uninitialize.vi"("error in (no error)"=w4, "Channel"=w2) -> ("error out"=w5:errorcluster)  [unwired: 8 in, 1 out]
  n2149 = call <vilib>:"Simple Error Handler.vi"("error code (no error:0)"=0, "error in (no error)"=w5) -> ()  [unwired: 3 in, 5 out]
  n2150 = call <vilib>:"Simple Error Handler.vi"("error code (no error:0)"=0, "error in (no error)"=w21) -> ()  [unwired: 3 in, 5 out]
